vi "Register4.vi"(4 "RF Out PWR":i8(slide)=3 scale=0.0..3.0, 5 "Aux Out PWR":i8(slide)=3 scale=0.0..3.0, 6 "RF out EN":bool=TRUE, 7 "AUX OUT EN":bool=TRUE, 8 "Mute till LD":bool, 9 "AUX OUT SEL":bool, 10 "Band Sel Div":i32=80, 11 "Out Divider":i32=1) -> (0 "HEX4":u32 format="%08x", 1 "Reg 4":bool[](array[boolean]))   [LabVIEW 2017]
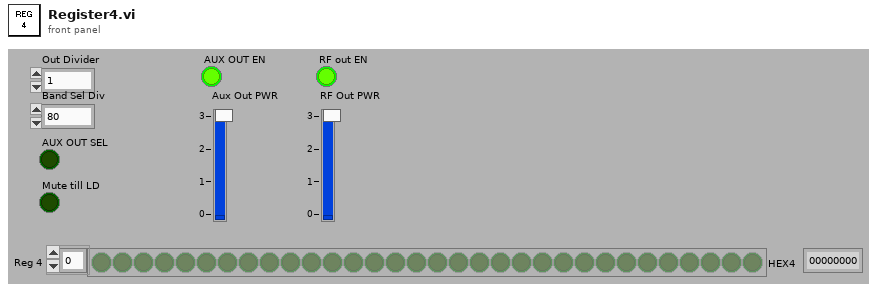
[diagram p1: front panel]
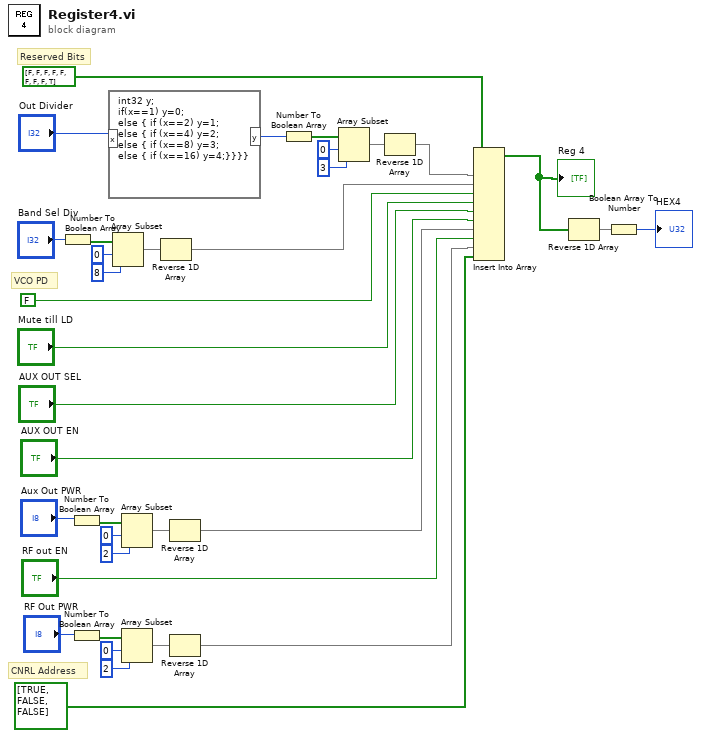
[diagram p0: block diagram]
diagram:
  # "VCO PD"
  # "Reserved Bits"
  # "CNRL Address"
  n1 = Number To Boolean Array(number="Band Sel Div") -> (Boolean array=w33:bool[])
  n2 = Number To Boolean Array(number="Aux Out PWR") -> (Boolean array=w14:bool[])
  n3 = Number To Boolean Array(number="RF Out PWR") -> (Boolean array=w10:bool[])
  n4 = formula code="int32 y;\nif(x==1) y=0;\nelse { if (x==2) y=1;\nelse { if (x==4) y=2;\nelse { if (x==8) y=3;\nelse { if (x==16) y=4;}}}}"("x"="Out Divider") -> ("y"=w2:i32)
  n5 = Array Subset(array=w33, index=0, length=8) -> (w32:bool[])
  n6 = Array Subset(array=w14, index=0, length=2) -> (w13:bool[])
  n7 = Array Subset(array=w10, index=0, length=2) -> (w9:bool[])
  n8 = Reverse 1D Array(array=w32) -> (reversed array=w22:bool[])
  n9 = Reverse 1D Array(array=w13) -> (reversed array=w6:bool[])
  n10 = Reverse 1D Array(array=w9) -> (reversed array=w4:bool[])
  n11 = Number To Boolean Array(number=w2) -> (Boolean array=w25:bool[])
  n12 = Array Subset(array=w25, index=0, length=3) -> (w24:bool[])
  n13 = Reverse 1D Array(array=w24) -> (reversed array=w23:bool[])
  n14 = Insert Into Array(array=bool[] [FALSE, FALSE, FALSE, FALSE, FALSE, FALSE, FALSE, FALSE, TRUE], new element #1=w23, new element #2=w22, new element #3=FALSE ("new element/subarray"), new element #4="Mute till LD", new element #5="AUX OUT SEL", new element #6="AUX OUT EN", new element #7=w6, new element #8="RF out EN", new element #9=w4, new element #10=bool[] [TRUE, FALSE, FALSE]) -> (w21:bool[])  [unwired: 1 in]
  "Reg 4" <- w21
  n15 = Reverse 1D Array(array=w21) -> (reversed array=w29:bool[])
  n16 = Boolean Array To Number(Boolean array=w29) -> (number=→"HEX4":u32)
